vi "TXMTest.vi"   [LabVIEW 2010]
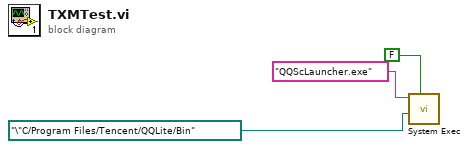
[diagram p0: block diagram]
diagram:
  n1 = call <vilib>:"System Exec.vi"("wait until completion? (T)"=FALSE, "working directory"=path "/\"C/Program Files/Tencent/QQLite/Bin", "command line"="QQScLauncher.exe") -> ()  [unwired: 5 in, 4 out]
